vi "Read Server RPC Methods.vi"(8 "error in (no error)":errorcluster, 11 "SignalGeneratorService in":refnum<class "ServiceManagementService.lvclass">) -> (0 "error out":errorcluster, 2 "Server RPC Methods":T1, 3 "SignalGeneratorService out":refnum<class "ServiceManagementService.lvclass">)   [LabVIEW 2020, in "Load Regulation.lvlib" / "ServiceManagementService.lvclass"]
uses:
  ServiceManagementService.lvclass
  typeDefs/Server gRPC UEs.ctl
  <vilib>/gRPC/LabVIEW gRPC Library/Server API/typeDefs/gRPCId Cluster.ctl
  <vilib>/gRPC/LabVIEW gRPC Library/Server API/typeDefs/grpcId.ctl
  ServiceManagementService.lvclass/ServiceManagementService.ctl
  <vilib>/gRPC/LabVIEW gRPC Library/gprc-lvsupport-release.lvlib
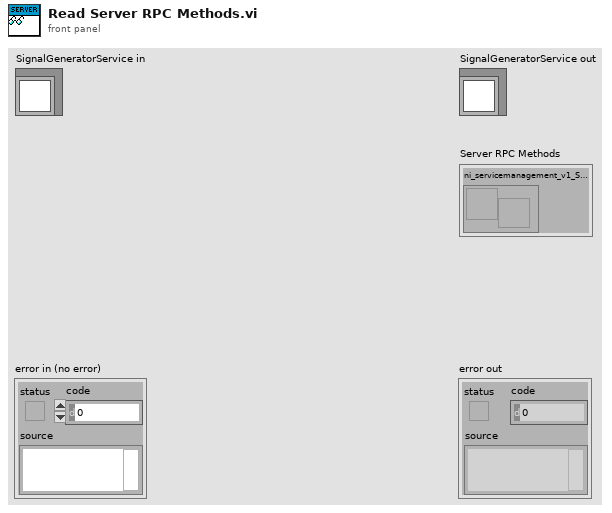
[diagram p1: front panel]
types:
  T1 = typedef "Load Regulation.lvlib/ServiceManagementService.lvclass/Server gRPC UEs.ctl" = cluster{"ni_servicemanagement_v1_ServiceManagementService_StopService gRPC UE":refnum<user-event>}
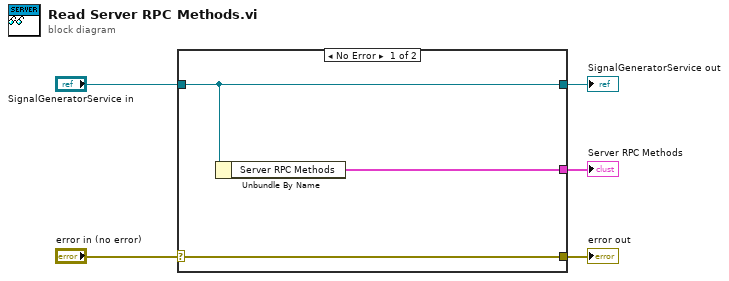
[diagram p0: block diagram]
diagram:
  n1 = case shown="No Error" "error in (no error)" {
    selector: "error in (no error)" -> [w8 w9]
    tunnel: [w8 w9] -> w4
    tunnel: [w7 w10] -> w2
    tunnel: "SignalGeneratorService in" -> [w7 w10]
    tunnel: [w6 _] -> w1
    frame No Error {
      n2 = Unbundle By Name(w7) -> ("Server RPC Methods"=w6:T1)
    }
    frame Error {
    }
  }
  "error out" <- w4
  "SignalGeneratorService out" <- w2
  "Server RPC Methods" <- w1
